vi "Fing Resonances.vi"() -> ()   [LabVIEW 2016]
uses:
  <vilib>/Analysis/3filter.llb/Filter Structure Type.ctl
  <vilib>/measure/macond.llb/IIR Filter for 1 Chan (CDB).vi
  <vilib>/Analysis/NI_AALPro.lvlib
  <vilib>/measure/NI_MAPro.lvlib
  <vilib>/Analysis/NI_AALBase.lvlib
  <vilib>/Analysis/NI_AAL_SigProc.lvlib
panel:
  in  "Fit?":bool
  in  "TDMS?":bool=TRUE
  in  "Deviations":dbl=1.0
  out "variance":dbl format="%.2p"
  out "standard deviation":dbl format="%.2p"
  out "Peak F":dbl
  in  "Points around peak":i32=100
  in  "Peak number":i32
  out "XY Graph 5":cluster{dbl[], dbl[]}(graph)
  in  "width":i32=100 min=3
  in  "optional IIR filter specifications":T1={"Lower PB"=100.0, "Upper PB"=0.0, "Lower SB"=200.0, "Upper SB"=0.0, "PB Gain"=-3.0, "SB Gain"=-60.0, "Scale"=TRUE} {"PB Gain" format="%0.2f"; "SB Gain" format="%0.2f"; "Lower SB" format="%0.2p"; "Upper SB" format="%0.2f"; "Lower PB" format="%0.2p"; "Upper PB" format="%0.2f"}
  in  "IIR filter specifications":T2={"Topology"=enum."Butterworth", "Type"=enum."Bandpass", "Order"=1, "Lower Fc"=1e-05, "Upper Fc"=0.01, "PB Ripple"=1.0, "SB Attenuation"=60.0} {"PB Ripple" format="%0.2f"; "SB Attenuation" format="%0.2f"; "Lower Fc" format="%0.2p"; "Upper Fc" format="%0.2p"}
  out "XY Graph 4":cluster{"Y":dbl[], dbl[]}(graph)
  out "XY Graph 3":cluster{"Y":dbl[], "Y":dbl[]}[](graph)
  out "XY Graph 2":cluster{"Y":dbl[], dbl[]}[](graph)
  out "XY Graph":cluster{"Y":dbl[], "Unwrapped Phase":dbl[]}[](graph)
  in  "File Path Control":path=path "D:/Data/RUS/Spectra/Ok spectra/300.00000K_175_555_2.10000V_0.00000T_May20-2015__09-37-18_001_052015.tdms"
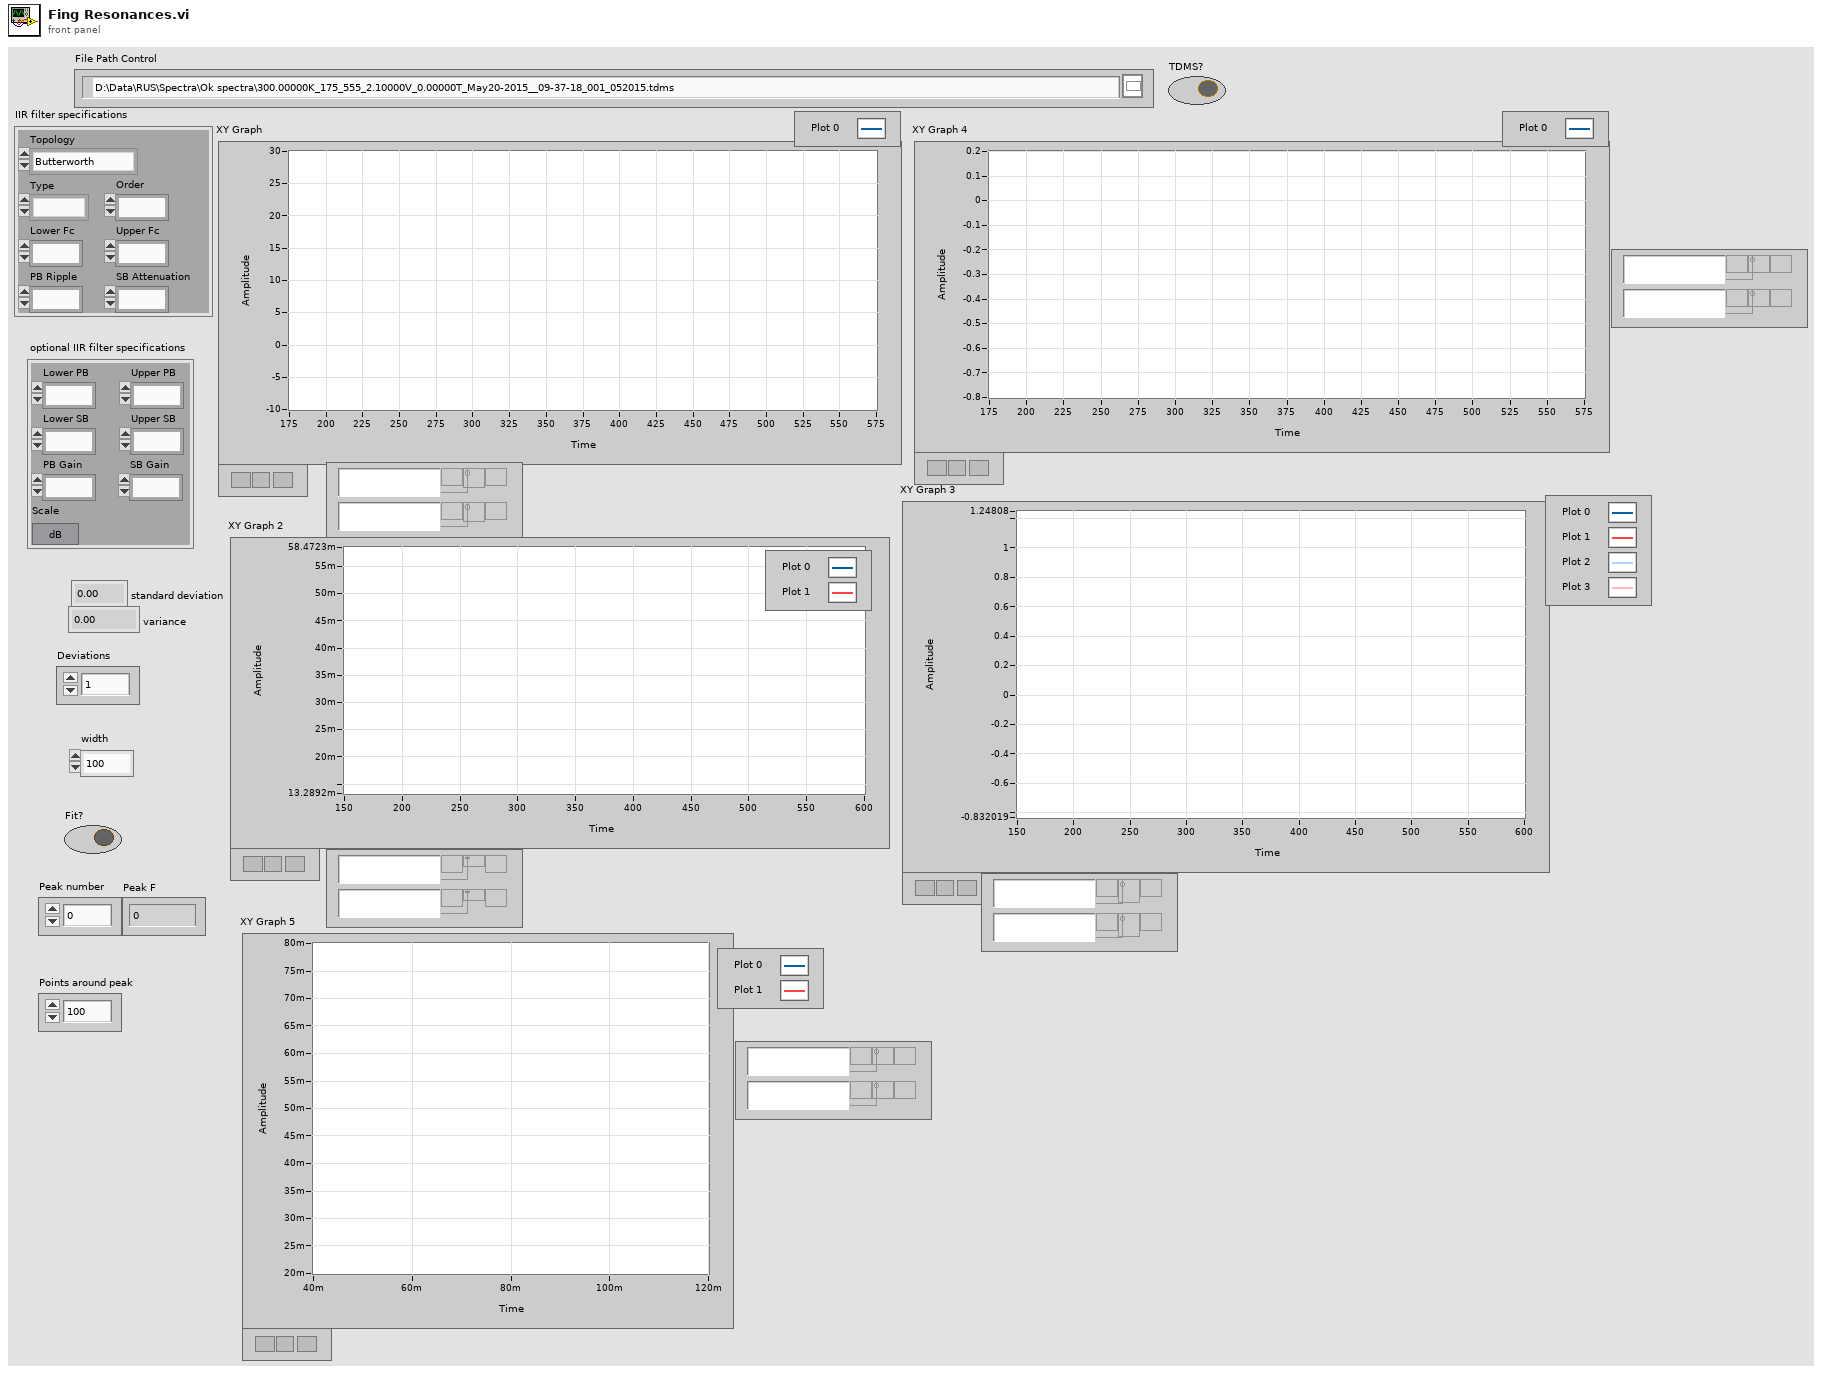
[diagram p1: front panel]
types:
  T1 = cluster{"Lower PB":dbl, "Upper PB":dbl, "Lower SB":dbl, "Upper SB":dbl, "PB Gain":dbl, "SB Gain":dbl, "Scale":bool}
  T2 = cluster{"Topology":enum16{"Off", "Butterworth", "Chebyshev", "Inverse Chebyshev", "Elliptic", "Bessel"}, "Type":enum16{"Lowpass", "Highpass", "Bandpass", "Bandstop"}, "Order":i32, "Lower Fc":dbl, "Upper Fc":dbl, "PB Ripple":dbl, "SB Attenuation":dbl}
  T3 = typedef "NI_AALBase.lvlib/Filter Structure Type.ctl" = u16
  T4 = enum16{"open", "open or create", "create or replace", "create", "open (read-only)"}
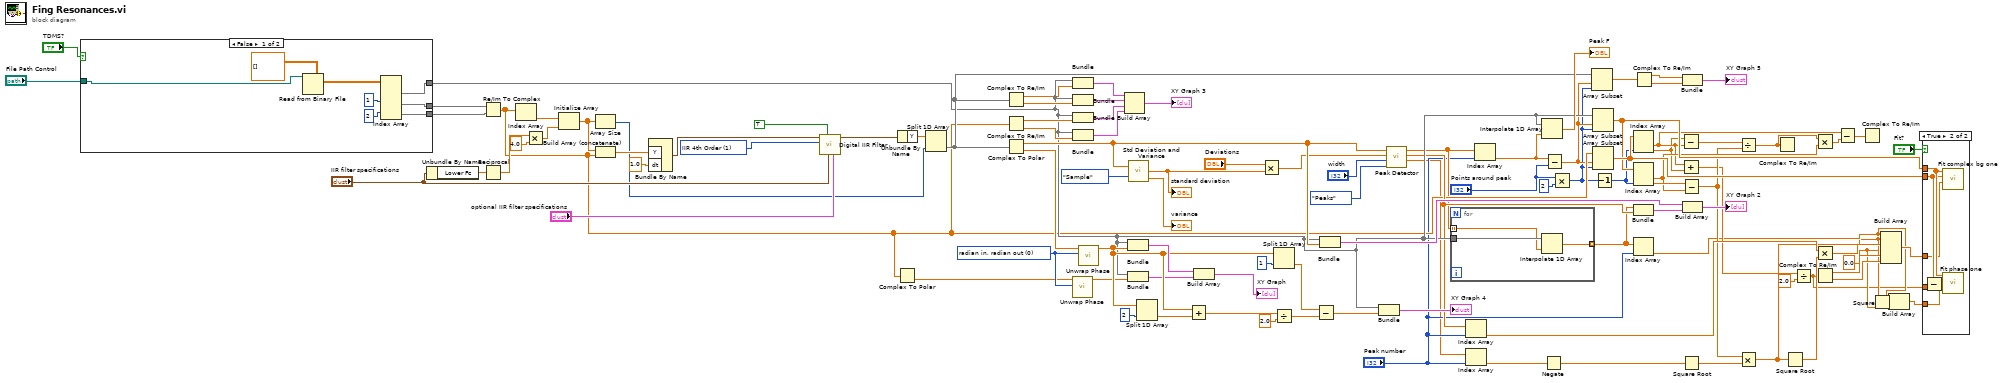
[diagram p0: block diagram]
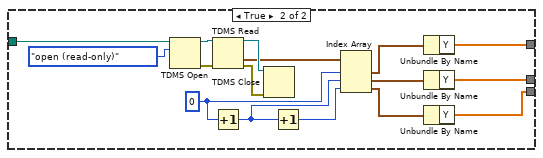
[diagram p3: hidden frame]
diagram:
  w4 = 0.0 ("element")
  w87 = T3 1 items=["IIR 2nd Order"=0, "IIR 4th Order"=1, "Auto Select"=10] ("filter structure option")
  w57 = 0 items=["radian in, radian out", "radian in, degree out", "degree in, degree out", "degree in, radian out"] ("phase unit")
  n1 = case shown="False" "TDMS?" {
    tunnel: "File Path Control" -> [w109 w129]
    tunnel: [w107 w117] -> w103
    tunnel: [w106 w116] -> w102
    tunnel: [w108 w114] -> w39
    frame False {
      n2 = Read from Binary File(5:dbl[][] [], 11:w109) -> (2:w112:dbl[][])  [unwired: 4 in, 3 out]
      n3 = Index Array(array=w112, index (row) #2=1 ("index (row)"), index (row) #3=2 ("index (row)")) -> (element #1=w108:dbl[], element #2=w107:dbl[], element #3=w106:dbl[])  [unwired: 4 in]
    }
    frame True {
      w122 = 0 ("index")
      n4 = TDMS Open(10:T4."open (read-only)" ("operation (0:open)"), 11:w129) -> (0:w126:errorcluster, 3:w127:refnum<k34>)  [unwired: 5 in]
      n5 = TDMS Read(0:w127, 11:w126) -> (4:w125:refnum<k34>, 10:w123:waveform(dbl)[], 15:w124:errorcluster)  [unwired: 6 in, 3 out]
      n6 = Increment(x=w122) -> (x+1=w120:i32)
      n7 = TDMS Close(8:w124, 11:w125) -> ()  [unwired: 2 out]
      n8 = Increment(x=w120) -> (x+1=w119:i32)
      n9 = Index Array(array=w123, index #1=w122, index #2=w120, index #3=w119) -> (element #1=w121:waveform(dbl), element #2=w115:waveform(dbl), element #3=w118:waveform(dbl))
      n10 = Unbundle By Name(w121) -> ("Y"=w114:dbl[])
      n11 = Unbundle By Name(w115) -> ("Y"=w117:dbl[])
      n12 = Unbundle By Name(w118) -> ("Y"=w116:dbl[])
    }
  }
  n13 = Unbundle By Name("IIR filter specifications") -> ("Lower Fc"=w51:dbl)
  n14 = Re/Im To Complex(1:w102, 2:w103) -> (0:w33:cdb[])
  n15 = Reciprocal(x=w51) -> (1/x=w50:dbl)
  n16 = Index Array(array=w33) -> (element=w48:cdb)  [unwired: 1 in]
  n17 = Multiply(x=w50, y=4.0) -> (x*y=w47:dbl)
  n18 = Initialize Array(w48, w47) -> (w45:cdb[])
  n19 = Array Size(array=w45) -> (size(s)=w43:i32)
  n20 = Build Array (concatenate)(w45, w33) -> (w46:cdb[])
  n21 = Bundle By Name("Y"=w46, "dt"=1.0) -> (w86:waveform(cdb))  [unwired: 1 in]
  n22 = call-poly <vilib>:"Digital IIR Filter.vi"("optional IIR filter specifications"="optional IIR filter specifications", "IIR filter specifications"="IIR filter specifications", "reset filter"=TRUE, "filter structure option"=w87, "signal in"=w86) -> ("signal out"=w85:waveform(cdb))  [unwired: 4 in, 2 out]
  n23 = Unbundle By Name(w85) -> ("Y"=w44:cdb[])
  n24 = Complex To Polar(r * e^(i*theta)=w33) -> (theta=w56:dbl[])  [unwired: 1 out]
  n25 = Split 1D Array(array=w44, index=w43) -> (second subarray=w42:cdb[])  [unwired: 1 out]
  n26 = Complex To Re/Im(x + iy=w42) -> (x=w82:dbl[], y=w80:dbl[])
  n27 = Complex To Re/Im(x + iy=w33) -> (x=w67:dbl[], y=w68:dbl[])
  n28 = Complex To Polar(r * e^(i*theta)=w42) -> (r=w64:dbl[], theta=w93:dbl[])
  n29 = call <vilib>:"Unwrap Phase.vi"("phase unit"=w57, "Phase"=w56) -> ("Unwrapped Phase"=w55:dbl[])  [unwired: 8 in, 1 out]
  n30 = Bundle("Y"=w39, w82) -> (w101:cluster{"Y":dbl[], dbl[]})  [unwired: 1 in]
  n31 = Bundle("Y"=w39, w80) -> (w100:cluster{"Y":dbl[], dbl[]})  [unwired: 1 in]
  n32 = Bundle("Y"=w39, w67) -> (w66:cluster{"Y":dbl[], dbl[]})  [unwired: 1 in]
  n33 = Bundle("Y"=w39, w68) -> (w65:cluster{"Y":dbl[], dbl[]})  [unwired: 1 in]
  n34 = call <vilib>:"Unwrap Phase.vi"("phase unit"=w57, "Phase"=w93) -> ("Unwrapped Phase"=w88:dbl[])  [unwired: 8 in, 1 out]
  n35 = Build Array(w101, w100, w66, w65) -> (→"XY Graph 3":cluster{"Y":dbl[], dbl[]}[])
  n36 = Bundle("Y"=w39, "Unwrapped Phase"=w88) -> (w104:cluster{"Y":dbl[], "Unwrapped Phase":dbl[]})  [unwired: 1 in]
  n37 = Bundle("Y"=w39, "Unwrapped Phase"=w55) -> (w53:cluster{"Y":dbl[], "Unwrapped Phase":dbl[]})  [unwired: 1 in]
  n38 = call <vilib>:"Std Deviation and Variance.vi"("X"=w64, "Weighting (Sample)"=enum16{"Sample", "Population"}."Sample") -> ("standard deviation"=w59:dbl, "variance"=→"variance":dbl)  [unwired: 1 out]
  "standard deviation" <- w59
  n39 = Split 1D Array(array=w88, index=2) -> (second subarray=w96:dbl[])  [unwired: 1 out]
  n40 = Add(x=w88, y=w96) -> (x+y=w95:dbl[])
  n41 = Build Array(w104, w53) -> (→"XY Graph":cluster{"Y":dbl[], "Unwrapped Phase":dbl[]}[])
  n42 = Multiply(x="Deviations", y=w59) -> (x*y=w60:dbl)
  n43 = Split 1D Array(array=w88, index=1) -> (second subarray=w89:dbl[])  [unwired: 1 out]
  n44 = Divide(x=w95, y=2.0) -> (x/y=w92:dbl[])
  n45 = Subtract(x=w89, y=w92) -> (x-y=w91:dbl[])
  n46 = Bundle("Y"=w39, w64) -> (w79:cluster{"Y":dbl[], dbl[]})  [unwired: 1 in]
  n47 = Bundle("Y"=w39, w91) -> (→"XY Graph 4":cluster{"Y":dbl[], dbl[]})  [unwired: 1 in]
  n48 = call <vilib>:"Peak Detector.vi"("peaks/valleys"=enum32{"Peaks", "Valleys"}."Peaks", "width"="width", "threshold"=w60, "X"=w64) -> ("2nd Derivatives"=w19:dbl[], "Amplitudes"=w37:dbl[], "Locations"=w21:dbl[])  [unwired: 3 in, 2 out]
  n49 = for {
    tunnel: w39 -> [w132]
    tunnel: w21 -> [w131] mode=indexing
    tunnel: [w130] -> w34 mode=indexing
    n50 = Interpolate 1D Array(1:w131, 2:w132) -> (0:w130:dbl)
  }
  n51 = Index Array(array=w37, index="Peak number") -> (element=w36:dbl)
  n52 = Index Array(array=w19, index="Peak number") -> (element=w18:dbl)
  n53 = Index Array(array=w21, index="Peak number") -> (element=w38:dbl)
  n54 = Interpolate 1D Array(1:w38, 2:w39) -> (0:→"Peak F":dbl)
  n55 = Negate(x=w18) -> (-x=w15:dbl)
  n56 = Subtract(x=w38, y="Points around peak") -> (x-y=w32:dbl)
  n57 = Multiply(x="Points around peak", y=2) -> (x*y=w30:i32)
  n58 = Array Subset(array=w42, index=w32, length=w30) -> (w40:cdb[])
  n59 = Array Subset(array=w39, index=w32, length=w30) -> (w28:dbl[])
  n60 = Array Subset(array=w33, index=w32, length=w30) -> (w31:cdb[])
  n61 = Decrement(x=w30) -> (x-1=w27:i32)
  n62 = Index Array(array=w31, index #2=w27) -> (element #1=w10:cdb, element #2=w9:cdb)  [unwired: 1 in]
  n63 = Index Array(array=w28, index #2=w27) -> (element #1=w23:dbl, element #2=w26:dbl)  [unwired: 1 in]
  n64 = Bundle(w34, "Amplitudes"=w37) -> (w75:cluster{dbl[], "Amplitudes":dbl[]})  [unwired: 1 in]
  n65 = Index Array(array=w34, index="Peak number") -> (element=w6:dbl)
  n66 = Complex To Re/Im(x + iy=w40) -> (x=w72:dbl[], y=w71:dbl[])
  n67 = Subtract(x=w9, y=w10) -> (x-y=w29:cdb)
  n68 = Add(x=w10, y=w9) -> (x+y=w8:cdb)
  n69 = Subtract(x=w26, y=w23) -> (x-y=w16:dbl)
  n70 = Square Root(x=w15) -> (sqrt(x)=w17:dbl)
  n71 = Bundle(w72, w71) -> (→"XY Graph 5":cluster{dbl[], dbl[]})  [unwired: 1 in]
  n72 = Build Array(w79, w75) -> (→"XY Graph 2":cluster{"Y":dbl[], "Amplitudes":dbl[]}[])
  n73 = Divide(x=w29, y=w16) -> (x/y=w24:cdb)
  n74 = Multiply(x=w16, y=w17) -> (x*y=w5:dbl)
  n75 = Complex To Re/Im(x + iy=w24) -> ()  [unwired: 2 out]
  n76 = Square Root(x=w5) -> (sqrt(x)=w11:dbl)
  n77 = Divide(x=w8, y=2.0) -> (x/y=w2:cdb)
  n78 = Multiply(x=w24, y=w23) -> (x*y=w22:cdb)
  n79 = Multiply(x=w36, y=w11) -> (x*y=w12:dbl)
  n80 = Complex To Re/Im(x + iy=w2) -> (x=w14:dbl, y=w13:dbl)
  n81 = Subtract(x=w10, y=w22) -> (x-y=w25:cdb)
  n82 = Complex To Re/Im(x + iy=w25) -> ()  [unwired: 2 out]
  n83 = Square(x=w5) -> (x^2=w1:dbl)
  n84 = Build Array(w6, w5, w12, w4, w14, w13) -> (w35:dbl[])
  n85 = Build Array(w6, w1, w4) -> (w3:dbl[])
  n86 = case shown="True" "Fit?" {
    tunnel: w31 -> [_ w137]
    tunnel: w28 -> [_ w138]
    tunnel: w35 -> [_ w136]
    tunnel: w3 -> [_ w135]
    tunnel: w2 -> [_ w133]
    frame False {
    }
    frame True {
      n87 = Subtract(x=w137, y=w133) -> (x-y=w134:cdb[])
      n88 = call "Fit complex bg one.vi"("Initial parameters"=w136, "Z"=w137, "X"=w138) -> ()  [unwired: 9 in]
      n89 = call "Fit phase one.vi"("Initial parameters"=w135, "Z"=w134, "X"=w138) -> ()  [unwired: 9 in]
    }
  }
